vi "写入亮度数据.vi"(0 "表格控件":string[][](table)) -> ()   [LabVIEW 2016]
doc: "本VI通过将表格写入Excel工作表说明利用OLE自动化VI的基本方式。"
panel:
  in  "Completion Task":u16(ring) caption="完成任务" items=["保持Excel打开", "关闭电子表格"]
  out "error out":errorcluster caption="错误输出"
  in  "error in (no error)":errorcluster caption="错误输入（无错误）"
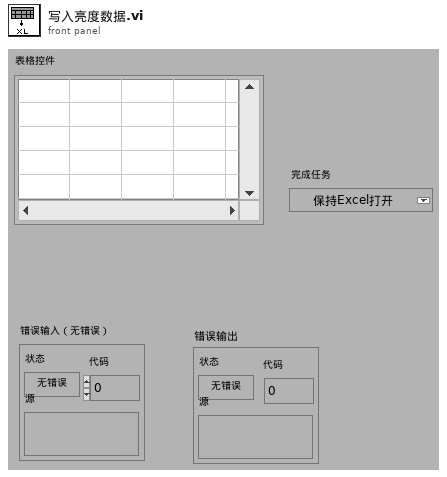
[diagram p1: front panel]
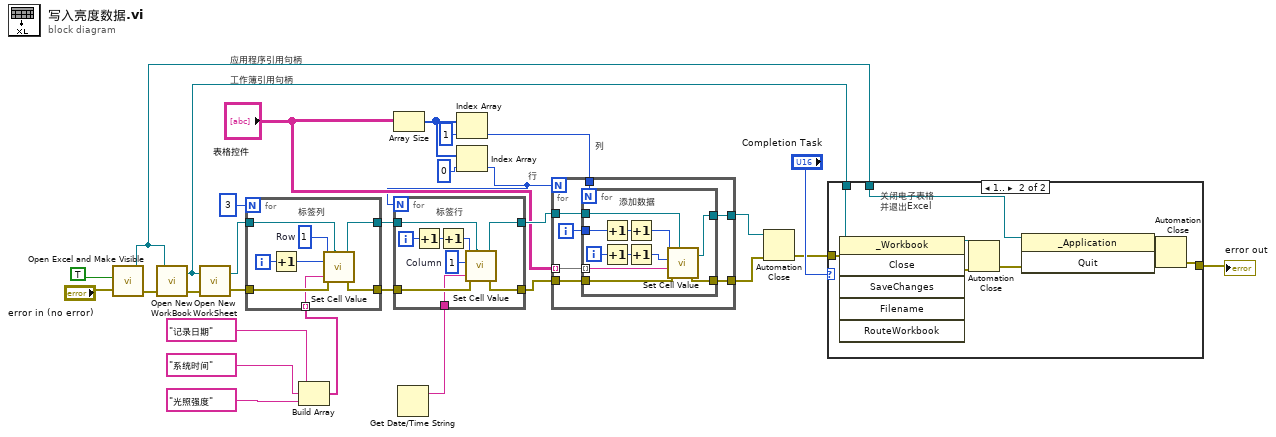
[diagram p0: block diagram]
diagram:
  # "列"
  # "行"
  # "工作簿引用句柄"
  # "应用程序引用句柄"
  n1 = call "Open Excel and Make Visible.vi"("error in (no error)"="error in (no error)", "Visible Boolean"=TRUE) -> ("error out"=w24:errorcluster, "Excel._Application"=w19:refnum<k7>)
  n2 = call "Open New  WorkBook.vi"("error in (no error)"=w24, "Excel._Application"=w19) -> ("error out"=w23:errorcluster, "Excel._Workbook"=w20:refnum<k7>)  [unwired: 1 out]
  n3 = call "Open New WorkSheet.vi"("error in (no error)"=w23, "Excel._Workbook"=w20) -> ("error out"=w14:errorcluster, "Excel._Worksheet"=w15:refnum<k7>)  [unwired: 1 out]
  n4 = Build Array("记录日期", "系统时间", "光照强度" ("元素")) -> (w13:string[])
  n5 = for {
    N: 3 -> [_]
    tunnel: w15 -> [w36]
    tunnel: w14 -> [w35]
    tunnel: [w34] -> w11
    tunnel: [w33] -> w9
    tunnel: w13 -> [w31] mode=indexing
    i -> [w37]
    w32 = 1  # Row
    # "标签列"
    n6 = Increment(x=w37) -> (x+1=w30:i32)
    n7 = call "Set Cell Value.vi"("Row"=w32, "Col"=w30, "Value"=w31, "error in (no error)"=w35, "Excel._Worksheet"=w36) -> ("Excel._Worksheet"=w33:refnum<k7>, "error out"=w34:errorcluster)
  }
  n8 = Array Size(array="表格控件") -> (size(s)=w29:i32[])
  n9 = Get Date/Time String() -> (date string=w7:string)  [unwired: 3 in, 1 out]
  n10 = Index Array(array=w29, index=1) -> (element=w22:i32)
  n11 = Index Array(array=w29, index=0) -> (element=w2:i32)
  n12 = for {
    N: w2 -> [_]
    tunnel: w9 -> [w42]
    tunnel: w11 -> [w41]
    tunnel: [w40] -> w10
    tunnel: [w39] -> w8
    tunnel: w7 -> [w38]
    i -> [w46]
    w44 = 1  # Column
    # "标签行"
    n13 = Increment(x=w46) -> (x+1=w45:i32)
    n14 = Increment(x=w45) -> (x+1=w43:i32)
    n15 = call "Set Cell Value.vi"("Row"=w43, "Col"=w44, "Value"=w38, "error in (no error)"=w41, "Excel._Worksheet"=w42) -> ("Excel._Worksheet"=w39:refnum<k7>, "error out"=w40:errorcluster)
  }
  n16 = for {
    N: w2 -> [_]
    tunnel: w8 -> [w53]
    tunnel: w10 -> [w51]
    tunnel: [w52] -> w18
    tunnel: "表格控件" -> [w50] mode=indexing
    tunnel: w22 -> [w49]
    tunnel: [w48] -> w16
    i -> [w47]
    n17 = for {
      N: w49 -> [_]
      tunnel: w53 -> [w60]
      tunnel: w51 -> [w59]
      tunnel: [w58] -> w52
      tunnel: w47 -> [w57]
      tunnel: w50 -> [w56] mode=indexing
      tunnel: [w55] -> w48
      i -> [w64]
      # "添加数据"
      n18 = Increment(x=w57) -> (x+1=w63:i32)
      n19 = Increment(x=w64) -> (x+1=w61:i32)
      n20 = Increment(x=w63) -> (x+1=w62:i32)
      n21 = Increment(x=w61) -> (x+1=w54:i32)
      n22 = call "Set Cell Value.vi"("Row"=w62, "Col"=w54, "Value"=w56, "error in (no error)"=w59, "Excel._Worksheet"=w60) -> ("Excel._Worksheet"=w55:refnum<k7>, "error out"=w58:errorcluster)
    }
  }
  n23 = Automation Close(3:w18, 5:w16) -> (0:w17:errorcluster)
  n24 = case shown="1.." "Completion Task" {
    tunnel: [w65 w66] -> w3
    tunnel: w20 -> [_ w74]
    tunnel: w19 -> [_ w70]
    tunnel: w17 -> [w65 w73]
    frame ..0 {
    }
    frame 1.. {
      # "关闭电子表格\n并退出Excel"
      n25 = invoke class="_Workbook" method="Close"(reference=w74, error in=w73) -> (reference out=w72:refnum<k7>, error out=w71:errorcluster)  [unwired: 4 in, 4 out]
      n26 = Automation Close(3:w71, 5:w72) -> (0:w69:errorcluster)
      n27 = invoke class="_Application" method="Quit"(reference=w70, error in=w69) -> (reference out=w67:refnum<k7>, error out=w68:errorcluster)  [unwired: 1 in, 1 out]
      n28 = Automation Close(3:w68, 5:w67) -> (0:w66:errorcluster)
    }
  }
  "error out" <- w3
